vi "Deadband.vi"(9 "Deadband":dbl, 11 "Input":dbl) -> (3 "Output":dbl)   [LabVIEW 2012]
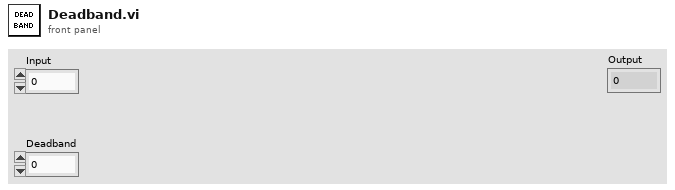
[diagram p1: front panel]
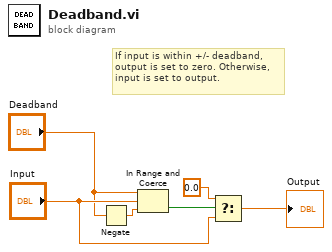
[diagram p0: block diagram]
diagram:
  # "If input is within +/- deadband, \noutput is set to zero. Otherwise,\ninput is set to output."
  n1 = Negate(x="Deadband") -> (-x=w2:dbl)
  n2 = In Range and Coerce(upper limit="Deadband", x="Input", lower limit=w2) -> (In Range?=w5:bool)  [unwired: 1 out]
  n3 = Select(t=0.0, s=w5, f="Input") -> (s? t:f=→"Output":dbl)
